vi "Handle Command.vi"(8 "error in (no error)":errorcluster, 10 "Parameters":string, 11 "Instrument in":refnum<class "Instrument.lvclass">) -> (0 "error out":errorcluster, 3 "Instrument out":refnum<class "Instrument.lvclass">)   [LabVIEW 2017, in "Instrument.lvlib" / "Instrument.lvclass"]
uses:
  Instrument.lvclass
  <vilib>/TSS/ACRObat Test Framework/Classes/Base Objects/Acrobat Base Object/Acrobat Base Object/Acrobat Base Object/typedefs/Command Cluster.ctl
  <vilib>/TSS/ACRObat Test Framework/Classes/Base Objects/Acrobat Base Object/Acrobat Base Object/Acrobat Base Object.lvclass
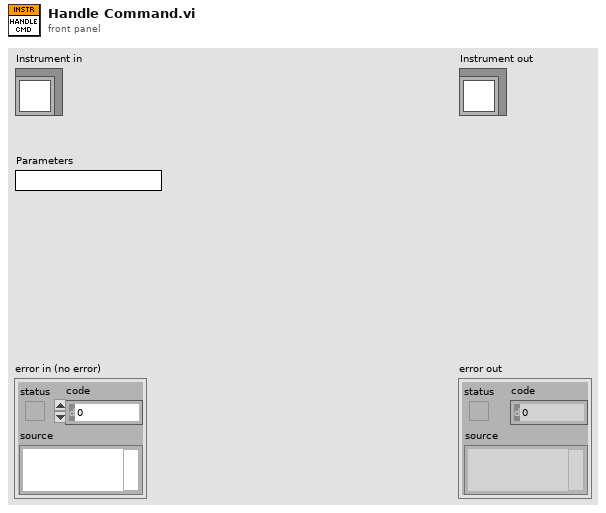
[diagram p1: front panel]
types:
  T1 = typedef "Acrobat Base Object.lvlib/Acrobat Base Object.lvclass/Command Cluster.ctl" = cluster{"Command":string, "Parameters":string}
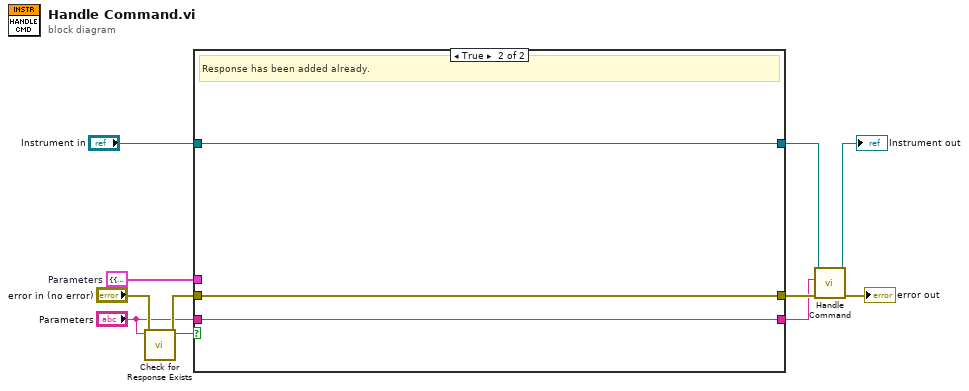
[diagram p0: block diagram]
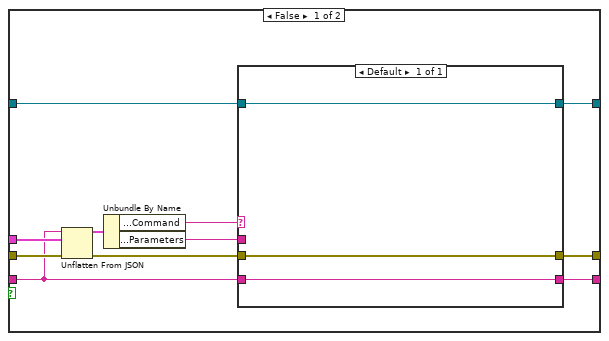
[diagram p2: hidden frame]
diagram:
  w6 = cluster{"Command Cluster":T1} {"Command Cluster"={"Command"="", "Parameters"=""}}  # Parameters
  n1 = call <vilib>:"Check for Response Exists.vi"("error in (no error)"="error in (no error)", "Parameters"="Parameters") -> ("error out"=w8:errorcluster, "Has Response"=w9:bool)  [unwired: 8 in]
  n2 = case shown="True" w9 {
    tunnel: "Instrument in" -> [w22 w28]
    tunnel: [w21 w28] -> w3
    tunnel: [w20 w26] -> w2
    tunnel: w8 -> [w19 w26]
    tunnel: w6 -> [w14 _]
    tunnel: "Parameters" -> [w13 w27]
    tunnel: [w12 w27] -> w1
    frame False {
      n3 = Unflatten From JSON(JSON string=w13, type and defaults=w14, error in (no error)=w19) -> (value=w17:cluster{"Command Cluster":T1}, error out=w18:errorcluster)  [unwired: 4 in]
      n4 = Unbundle By Name(w17) -> ("Command Cluster.Command"=w16:string, "Command Cluster.Parameters"=w15:string)
      n5 = case shown="Default" w16 {
        tunnel: w22 -> [w25]
        tunnel: [w25] -> w21
        tunnel: w18 -> [w24]
        tunnel: [w24] -> w20
        tunnel: w15 -> [_]
        tunnel: w13 -> [w23]
        tunnel: [w23] -> w12
        frame Default {
        }
      }
    }
    frame True {
      # "Response has been added already."
    }
  }
  n6 = call-parent "Handle Command.vi"("error in (no error)"=w2, "Parameters"=w1, "Instrument in"=w3) -> ("error out"=→"error out":errorcluster, "Instrument out"=→"Instrument out":refnum<class "Instrument.lvclass">)  [unwired: 7 in]
